vi "Sequence_from_name.vi"(10 "Sequence name":string, 11 "Sequences":T2(array[cluster])) -> (3 "Sequence":T1)   [LabVIEW 2016]
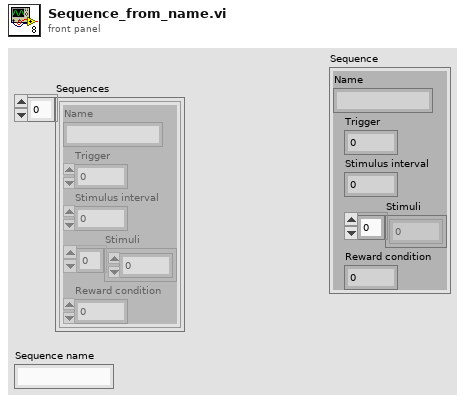
[diagram p1: front panel]
types:
  T1 = cluster{"Name":string, "Trigger":u16, "Stimulus interval":dbl, "Stimuli":i32[], "Reward condition":u16}
  T2 = cluster{"Name":string, "Trigger":u16, "Stimulus interval":dbl, "Stimuli":i32[], "Reward condition":u16}[]
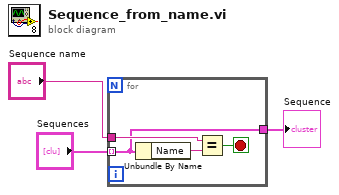
[diagram p0: block diagram]
diagram:
  n1 = for {
    tunnel: "Sequences" -> [w4] mode=indexing
    tunnel: "Sequence name" -> [w6]
    tunnel: [w4] -> w1
    stop <- w5 stop-if-true
    n2 = Unbundle By Name(w4) -> ("Name"=w7:string)
    n3 = Equal?(x=w6, y=w7) -> (x = y?=w5:bool)
  }
  "Sequence" <- w1
